vi "InitConfigFile.vi"(8 "error in (no error)":errorcluster caption="에러 입력(에러 없음)", 11 "init 파일 경로":string) -> (0 "error out":errorcluster caption="에러 출력", 3 "Config File Data":T1)   [LabVIEW 2018]
uses:
  <vilib>/Utility/config.llb/NI_LVConfig.lvlib
  <vilib>/Utility/config.llb/Read Key (String).vi
  ConfigFileData.ctl
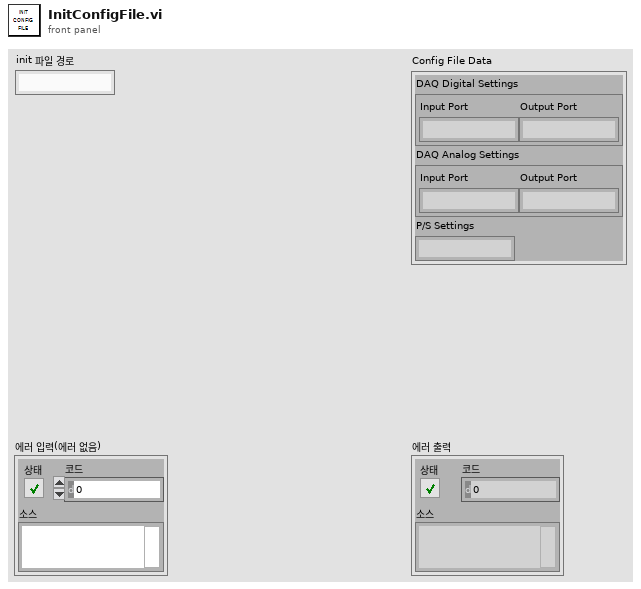
[diagram p1: front panel]
types:
  T1 = typedef "ConfigFileData.ctl" = cluster{"DAQ Digital Settings":cluster{"Input Port":string, "Output Port":string}, "DAQ Analog Settings":cluster{"Input Port":string, "Output Port":string}, "P/S Settings":string}
  T2 = typedef "NI_LVConfig.lvlib/Config Data RefNum.ctl" = refnum<k1>
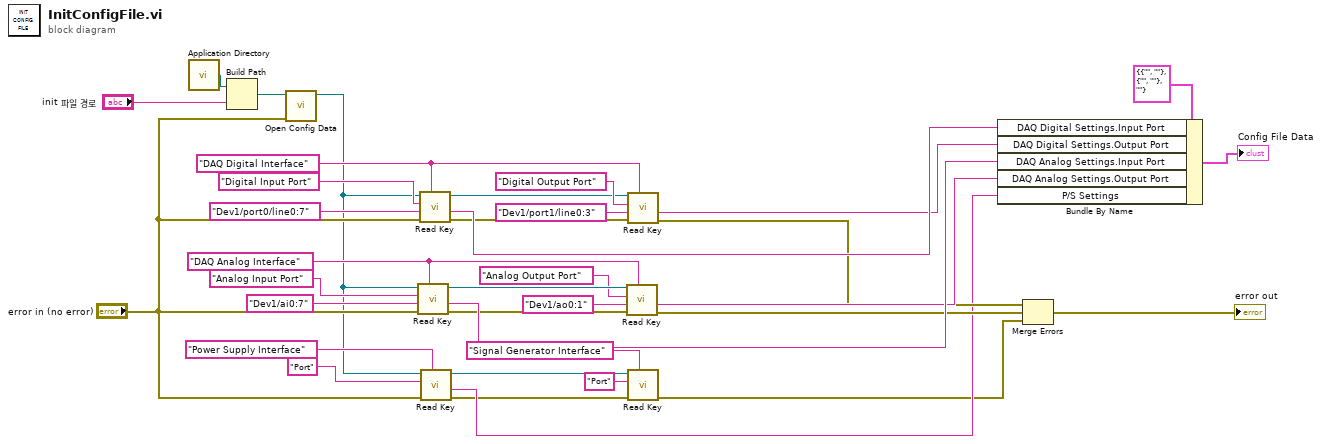
[diagram p0: block diagram]
diagram:
  w22 = "DAQ Analog Interface" ("section")
  w30 = "DAQ Digital Interface" ("section")
  n1 = call <vilib>:"Application Directory.vi"() -> ("Application Directory"=w36:path)
  n2 = Build Path(base path=w36, name or relative path="init 파일 경로") -> (appended path=w35:path)
  n3 = call <vilib>:"Open Config Data.vi"("error in (no error)"="error in (no error)", "configuration file path"=w35) -> ("refnum"=w6:T2)  [unwired: 7 in, 2 out]
  n4 = call-poly <vilib>:"Read Key.vi"("section"=w22, "error in (no error)"="error in (no error)", "default value"="Dev1/ai0:7", "key"="Analog Input Port", "refnum"=w6) -> ("error out"=w14:errorcluster, "value"=w17:string, "refnum out"=w23:T2)  [unwired: 3 in, 1 out]
  n5 = call-poly <vilib>:"Read Key.vi"("section"=w30, "error in (no error)"="error in (no error)", "default value"="Dev1/port0/line0:7", "key"="Digital Input Port", "refnum"=w6) -> ("error out"=w15:errorcluster, "value"=w25:string, "refnum out"=w28:T2)  [unwired: 3 in, 1 out]
  n6 = call-poly <vilib>:"Read Key.vi"("section"="Power Supply Interface", "error in (no error)"="error in (no error)", "key"="Port", "refnum"=w6) -> ("error out"=w2:errorcluster, "value"=w7:string, "refnum out"=w5:T2)  [unwired: 4 in, 1 out]
  n7 = call-poly <vilib>:"Read Key.vi"("section"=w22, "error in (no error)"=w14, "default value"="Dev1/ao0:1", "key"="Analog Output Port", "refnum"=w23) -> ("error out"=w12:errorcluster, "value"=w16:string)  [unwired: 3 in, 2 out]
  n8 = call-poly <vilib>:"Read Key.vi"("section"=w30, "error in (no error)"=w15, "default value"="Dev1/port1/line0:3", "key"="Digital Output Port", "refnum"=w28) -> ("error out"=w13:errorcluster, "value"=w24:string)  [unwired: 3 in, 2 out]
  n9 = call-poly <vilib>:"Read Key.vi"("section"="Signal Generator Interface", "error in (no error)"=w2, "key"="Port", "refnum"=w5) -> ("error out"=w1:errorcluster)  [unwired: 4 in, 3 out]
  n10 = Bundle By Name(cluster=T1 {"DAQ Digital Settings"={"Input Port"="", "Output Port"=""}, "DAQ Analog Settings"={"Input Port"="", "Output Port"=""}, "P/S Settings"=""} ("Config File Data"), "DAQ Digital Settings.Input Port"=w25, "DAQ Digital Settings.Output Port"=w24, "DAQ Analog Settings.Input Port"=w17, "DAQ Analog Settings.Output Port"=w16, "P/S Settings"=w7) -> (→"Config File Data":T1)
  n11 = Merge Errors(w13, w12, w1) -> (→"error out":errorcluster)
